vi "Eval y=f(x) Prep1.vi"(0 "end":dbl format="%.2f", 1 "number of points":u32, 2 "start":dbl format="%.2f", 3 "List of variables":i32[](array[numeric]), 5 "formula":string) -> (4 "random summand":dbl format="%.2f", 6 "Parsed Formula":cluster{"Table":i32[][], "Y Values":dbl[]} {"Y Values" format="%.2f"}, 7 "points":dbl[](array[numeric]) format="%.2f", 8 "points II":dbl[](array[numeric]) format="%.2f", 9 "points I":dbl[](array[numeric]) format="%.2f")   [LabVIEW 2014, in "NI_Gmath.lvlib"]
uses:
  NI_Gmath.lvlib
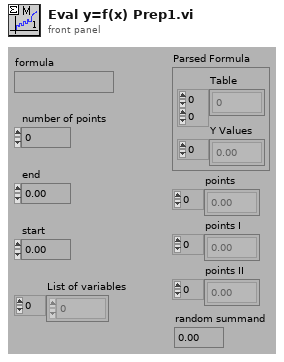
[diagram p1: front panel]
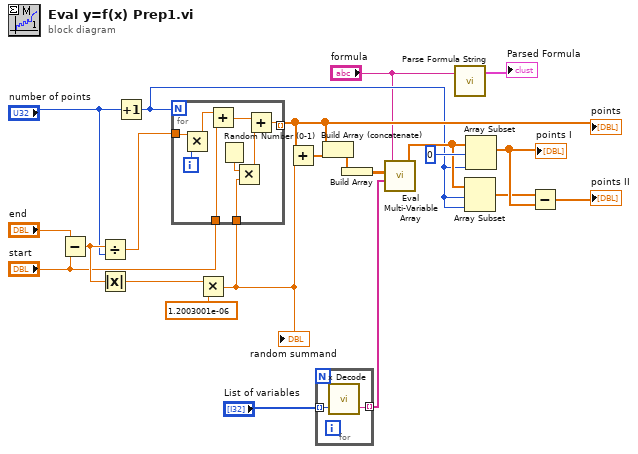
[diagram p0: block diagram]
diagram:
  n1 = Subtract(x="end", y="start") -> (x-y=w18:dbl)
  n2 = Divide(x=w18, y="number of points") -> (x/y=w17:dbl)
  n3 = Absolute Value(x=w18) -> (abs(x)=w10:dbl)
  n4 = Increment(x="number of points") -> (x+1=w7:u32)
  n5 = Multiply(x=w10, y=1.2003001e-06) -> (x*y=w6:dbl)
  "random summand" <- w6
  n6 = for {
    N: w7 -> [_]
    tunnel: w17 -> [w31]
    tunnel: "start" -> [w28]
    tunnel: [w23] -> w9 mode=indexing
    tunnel: w6 -> [w25]
    i -> [w30]
    n7 = Multiply(x=w31, y=w30) -> (x*y=w29:dbl)
    n8 = Add(x=w29, y=w28) -> (x+y=w27:dbl)
    n9 = Random Number (0-1)() -> (number: 0 to 1=w26:dbl)
    n10 = Multiply(x=w26, y=w25) -> (x*y=w24:dbl)
    n11 = Add(x=w27, y=w24) -> (x+y=w23:dbl)
  }
  "points" <- w9
  n12 = Add(x=w9, y=w6) -> (x+y=w16:dbl[])
  n13 = for {
    tunnel: "List of variables" -> [w33] mode=indexing
    tunnel: [w32] -> w21 mode=indexing
    n14 = call "x Decode.vi"("number"=w33) -> ("x string"=w32:string)  [unwired: 1 in, 1 out]
  }
  n15 = Build Array (concatenate)(w9, w16) -> (w15:dbl[])
  n16 = Build Array(w15) -> (w20:dbl[][])
  n17 = call "Eval Multi-Variable Array.vi"("Variables"=w21, "X Values"=w20, "formula"="formula") -> ("Y Values"=w13:dbl[])  [unwired: 1 in, 1 out]
  n18 = call "Parse Formula String.vi"("formula"="formula") -> ("Parsed Formula"=→"Parsed Formula":cluster{"Table":i32[][], "Y Values":dbl[]})  [unwired: 1 in, 1 out]
  n19 = Array Subset(array=w13, index=w7, length=w7) -> (w12:dbl[])
  n20 = Array Subset(array=w13, index=0, length=w7) -> (w19:dbl[])
  "points I" <- w19
  n21 = Subtract(x=w12, y=w19) -> (x-y=→"points II":dbl[])
